vi "Add Event Details of students.vi"() -> ()   [LabVIEW 2014]
panel:
  in  "Event Name":string="004"
  out "Match Found":bool
  in  "Radio Buttons":T1(radio)
  in  "Round Details":string[](array[string])
  in  "Event Number":i16
  in  "Search Reg No":string[](array[string])
  # "New Event Name :"
  # "Event Number  :"
  # "Search Reg Numbers"
  # "Round Details"
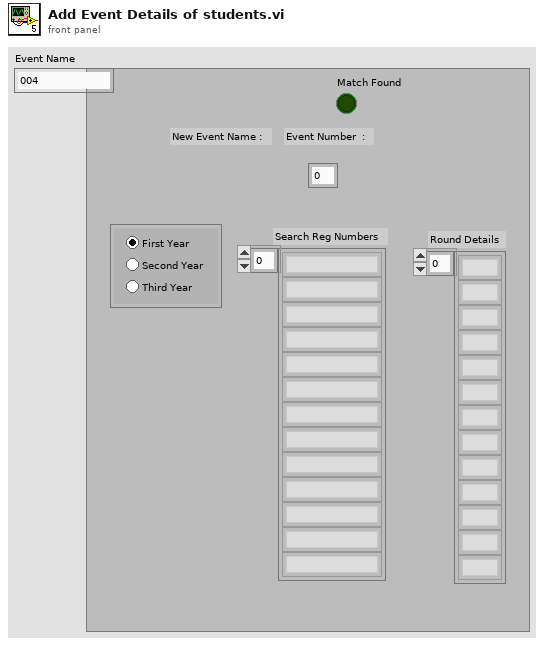
[diagram p1: front panel]
types:
  T1 = enum32{"Radio Selection 1", "Radio Selection 2", "Radio Selection 3"}
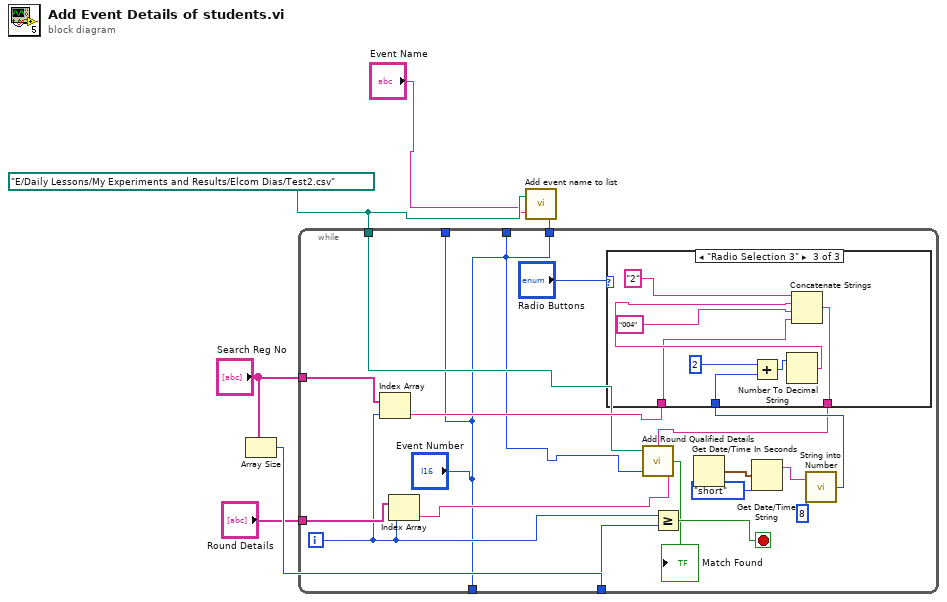
[diagram p0: block diagram]
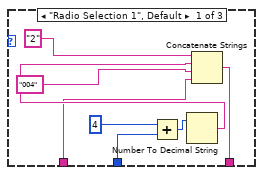
[diagram p2: hidden frame]
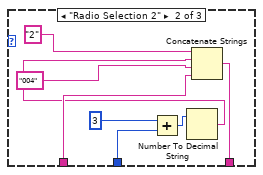
[diagram p3: hidden frame]
diagram:
  w3 = path "E:/Daily Lessons/My Experiments and Results/Elcom Dias/Test2.csv" ("file path (dialog if empty)")
  n1 = Array Size(array="Search Reg No") -> (size(s)=w5:i32)
  n2 = while {
    tunnel: "Search Reg No" -> [w23]
    tunnel: w5 -> [w21]
    tunnel: "Round Details" -> [w20]
    tunnel: w3 -> [w11]
    tunnel: ["Event Number"] -> _
    tunnel: ["Event Number"] -> _
    tunnel: ["Event Number"] -> _
    tunnel: ["Event Number"] -> w1
    i -> [w19]
    stop <- w22 stop-if-true
    n3 = Index Array(array=w23, index=w19) -> (element=w17:string)
    n4 = Index Array(array=w20, index=w19) -> (element=w9:string)
    n5 = Greater Or Equal?(x=w19, y=w21) -> (x >= y?=w22:bool)
    n6 = Get Date/Time In Seconds() -> (seconds since 1Jan1904=w16:timestamp)
    n7 = Get Date/Time String(date format (0)=enum16{"short", "long", "abbreviated"}."short", seconds (now)=w16) -> (date string=w12:string)  [unwired: 1 in, 1 out]
    n8 = call "String into Number.vi"("initial scan location"=u32 8, "String"=w12) -> ("output 1"=w14:i32)
    n9 = case shown="\"Radio Selection 3\"" "Radio Buttons" {
      tunnel: w17 -> [w25 w34 w40]
      tunnel: w14 -> [w30 w33 w42]
      tunnel: [w24 w35 w43] -> w10
      frame "Radio Selection 1", Default {
        n10 = Add(x=4, y=w30) -> (x+y=w28:i32)
        n11 = Number To Decimal String(number=w28) -> (decimal integer string=w27:string)  [unwired: 1 in]
        n12 = Concatenate Strings("2" ("string"), w27, "004" ("string"), w25) -> (w24:string)
      }
      frame "Radio Selection 2" {
        n13 = Add(x=3, y=w33) -> (x+y=w37:i32)
        n14 = Number To Decimal String(number=w37) -> (decimal integer string=w32:string)  [unwired: 1 in]
        n15 = Concatenate Strings("2" ("string"), w32, "004" ("string"), w34) -> (w35:string)
      }
      frame "Radio Selection 3" {
        n16 = Add(x=2, y=w42) -> (x+y=w45:i32)
        n17 = Number To Decimal String(number=w45) -> (decimal integer string=w41:string)  [unwired: 1 in]
        n18 = Concatenate Strings("2" ("string"), w41, "004" ("string"), w40) -> (w43:string)
      }
    }
    n19 = call "Add Round Qualified Details.vi"("Qualified for round"=w9, "Search Element"=w10, "Event Number"="Event Number", "file path (dialog if empty)"=w11) -> ("Match Found"=→"Match Found":bool)
  }
  n20 = call "Add event name to list.vi"("Event Number"=w1, "Event Name"="Event Name", "file path (dialog if empty)"=w3) -> ()
